vi "Set command buttons blinking.vi"(7 "Go To Ref":refnum<vi>, 8 "error in (no error)":errorcluster, 9 "Values":T1[](array[typedef]), 10 "In Ref":refnum<vi>, 11 "Out Ref":refnum<vi>) -> (0 "error out":errorcluster)   [LabVIEW 2011]
uses:
  Measurments Handling/Status Digitalish.ctl
  Tool/Variable List Tool Digital.ctl
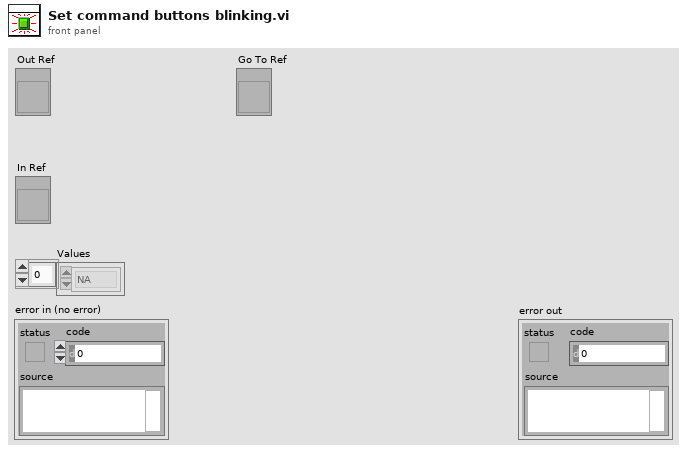
[diagram p1: front panel]
types:
  T1 = typedef "Status Digitalish.ctl" = enum16{"NA", "False", "True"}
  T2 = typedef "Variable List Tool Digital.ctl" = enum16{"Tool Error Controller", "Tool Stopped Controller", "Tool Relay 1", "Tool Relay 2", "Tool Both Relays", "Tool node Pressure 1", "Tool Error Pressure 1", "Tool Stopped Pressure 1", "Tool node Pressure 2", "Tool Error Pressure 2", "Tool Stopped Pressure 2", "Tool node Solenoid", "Tool Error Solenoid", "Tool Stopped Solenoid", "Tool Solenoid 1", "Tool Solenoid 2", "Tool Solenoid 3", "Tool node PSU", "Tool Error PSU", "Tool Stopped PSU", "Upper Tension Sub", "Tool Error Upper Tension Sub", "Tool Stopped Upper Tension Sub", "Lower Tension Sub", "Tool Error Lower Tension Sub", "Tool Stopped Lower Tension Sub", "Stroke Target seeking", "Stroke Moving Out", "Stroke Moving Inn", "Stroke valves set for Out", "Stroke valves set for In", "Stroke In (force)", "Stroke Out (force)", "Stroke Force decreasing(in)", "Stroke Force decreasing(out)", "Stroke Force change not correct", "Stroke SLIPS established P1", "Stroke SLIPS established P2", "Stroke SLIPS established", "Stroke Pressure Monitor Ongoing", "Stroke Pressure Monitor Ending ", "Tool Stroke enable Valve", "Tool Stroke direction Valve", "Tool Anchor Valve", "Stroker Var19 - Reserved", "Stroker Var20 - Reserved", "Stroker Var21 - Reserved", "Stroker Var22 - Reserved", "Stroker Var23 - Reserved", "Stroker Var24 - Reserved", "Tractor Var1 - Reserved", "Tractor Var2 - Reserved", "Tractor Var3 - Reserved", "Tractor Var4 - Reserved", "Tractor Var5 - Reserved", "Tractor Var6 - Reserved", "Tractor Var7 - Reserved", "Tractor Var8 - Reserved", "Oil filling mode", "Mill Bit Direction", "Position control", "Anchor", "Driller Var5 - Reserved", "Driller Var6 - Reserved", "Driller Var7 - Reserved", "Driller Var8 - Reserved"}
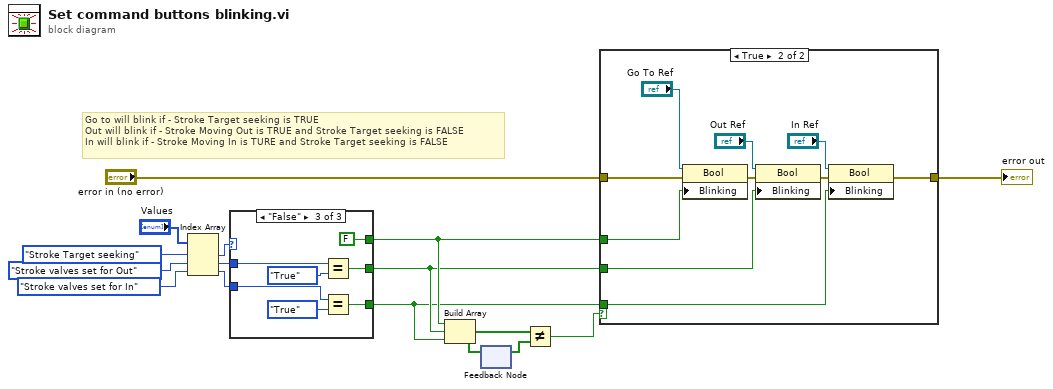
[diagram p0: block diagram]
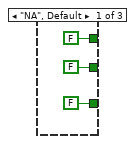
[diagram p3: hidden frame]
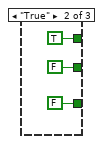
[diagram p4: hidden frame]
diagram:
  # "Go to will blink if - Stroke Target seeking is TRUE\nOut will blink if - Stroke Moving Out is TRUE and Stroke Target seeking is FALSE\nIn will blink if - Stroke Moving In is TURE and Stroke Target seeking is FALSE"
  n1 = Index Array(array="Values", index #1=Variable_List_Tool_Digital."Stroke Target seeking", index #2=Variable_List_Tool_Digital."Stroke valves set for Out", index #3=Variable_List_Tool_Digital."Stroke valves set for In") -> (element #1=w14:T1, element #2=w13:T1, element #3=w12:T1)
  n2 = case shown="\"False\"" w14 {
    tunnel: [FALSE ("Blinking") TRUE ("Blinking") FALSE ("Blinking")] -> w9
    tunnel: [FALSE ("Blinking") FALSE ("Blinking") w23] -> w8
    tunnel: [FALSE ("Blinking") FALSE ("Blinking") w24] -> w7
    tunnel: w13 -> [_ _ w28]
    tunnel: w12 -> [_ _ w25]
    frame "NA", Default {
    }
    frame "True" {
    }
    frame "False" {
      n3 = Equal?(x=w28, y=Status_Digitalish."True") -> (x = y?=w23:bool)
      n4 = Equal?(x=w25, y=Status_Digitalish."True") -> (x = y?=w24:bool)
    }
  }
  n5 = Build Array(w9, w8, w7) -> (w5:bool[])
  n6 = feedback-in #1(w5) -> ()
  n7 = feedback #1() -> (w6:bool[])  [unwired: 1 in]
  n8 = Not Equal?(x=w5, y=w6) -> (x != y?=w4:bool)
  n9 = case shown="True" w4 {
    tunnel: "error in (no error)" -> [w29 w37]
    tunnel: [w29 w36] -> w10
    tunnel: w9 -> [_ w32]
    tunnel: w8 -> [_ w31]
    tunnel: w7 -> [_ w30]
    frame False {
    }
    frame True {
      n10 = property on="Property Node" class="Bool"(reference="Go To Ref", error in=w37, "Blinking"=w32) -> (error out=w39:errorcluster)  [unwired: 1 out]
      n11 = property on="Property Node" class="Bool"(reference="Out Ref", error in=w39, "Blinking"=w31) -> (error out=w38:errorcluster)  [unwired: 1 out]
      n12 = property on="Property Node" class="Bool"(reference="In Ref", error in=w38, "Blinking"=w30) -> (error out=w36:errorcluster)  [unwired: 1 out]
    }
  }
  "error out" <- w10
